vi "MLP_forwardpass_MLP2.vi"(11 "Array in":fxp<+/-,64,35>[](array[numeric])=[0.0, 0.0, 0.0, 0.0, 0.0, 0.0, 0.0, 0.0, 0.0, 0.0]) -> (3 "Numeric":fxp<+/-,32,16>)   [LabVIEW 2020]
uses:
  <vilib>/rvi/DataTransferAndStorage/Container/Common/niFpgaContainerExecOnDevCompGetState.vi
  <vilib>/rvi/Emulation/niFpgaEmulationIsFPGAContextNoSignature.vi
  <vilib>/rvi/DataTransferAndStorage/Container/Common/niFpgaContainerGetUniqueNameForEmu.vi
  <vilib>/rvi/Memory/Memory_Emulation/niFpgaMemoryEmulationCacheClearOnFirstRun.vi
  <vilib>/rvi/Memory/Memory_Emulation/nirvimemoryEmulationManagerCache_MakeExclusive.vi
  <vilib>/rvi/Memory/Memory_Emulation/niFpgaMemoryEmulationValidateCache.vi
  <vilib>/rvi/Memory/Memory_Emulation/nirvimemoryEmulationManagerCache_InsertValue.vi
  <vilib>/Utility/error.llb/Clear Errors.vi
  <vilib>/rvi/Memory/Memory_Emulation/nirvimemoryEmulationManagerCache_ReleaseExclusive.vi
  <vilib>/rvi/Memory/Memory_Emulation/nirvimemoryEmulationManagerCache_GetValue.vi
  <vilib>/rvi/Memory/Memory_Emulation/nirvimemoryEmulationManagerCache_SetValue.vi
  <vilib>/rvi/Emulation/niFpgaProcessEmulError.vi
  <vilib>/rvi/Emulation/niFpgaSctlEmulationGetInTimedLoop.vi
  <vilib>/rvi/errors/nirviReportUnexpectedCaseInternalError (U32).vi
  <vilib>/rvi/Emulation/niFpgaSctlEmulationResourceMgr.vi
  <vilib>/rvi/DataTransferAndStorage/Container/XNode/niFpgaContainer.xnode
  <vilib>/rvi/DataTransferAndStorage/Register/Emulation/niFpgaRegisterEmulationRefIn.vi
  <vilib>/rvi/Memory/Memory_Emulation/niFpgaMemoryEmulationRefIn.vi
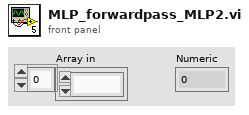
[diagram p1: front panel]
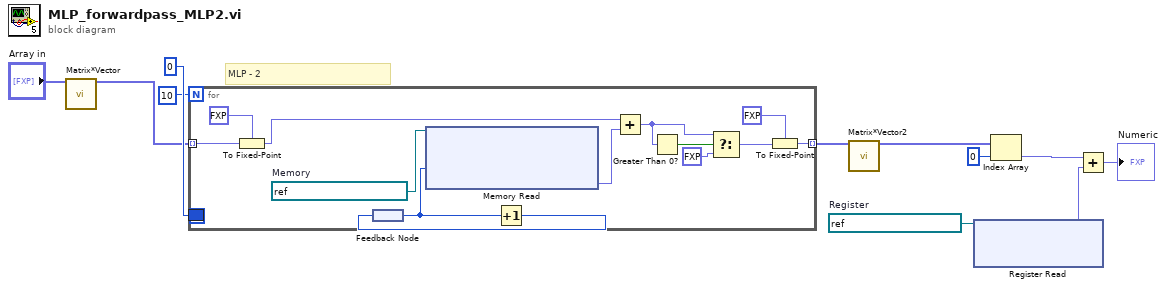
[diagram p0: block diagram]
diagram:
  w6 = refnum<k21> "Register-MLP_2_B_1"  # Register
  # "MLP - 2"
  n1 = call "Matrix*Vector"("Vector b"="Array in") -> ("Vector c"=w4:fxp<+/-,64,36>[])  [unwired: 10 in]
  n2 = for {
    N: 10 -> [_]
    tunnel: w4 -> [w15] mode=indexing
    tunnel: [w12] -> w3 mode=indexing
    border: u32 0 ("Timeout") -> [_]
    w19 = refnum<k21> "Memory-MLP_2_B_0"  # Memory
    n3 = To Fixed-Point(fixed-point type=fxp<+/-,32,16> 0.0 ("f"), number=w15) -> (fixed-point=w20:fxp<+/-,32,16>)
    n4 = feedback #1() -> (w18:u32)
    n5 = xnode ("Memory Read")("Address"=w18, "Memory In"=w19) -> ("Data"=w16:fxp<+/-,32,16>)  [unwired: 1 out]
    n6 = Increment(x=w18) -> (x+1=w17:u32)
    n7 = feedback-in #1(w17) -> ()
    n8 = Add(x=w20, y=w16) -> (x+y=w22:fxp<+/-,33,17>)
    n9 = Greater Than 0?(x=w22) -> (x > 0?=w24:bool)
    n10 = Select(t=w22, s=w24, f=fxp<+/-,33,17> 0.0) -> (s? t:f=w13:fxp<+/-,33,17>)
    n11 = To Fixed-Point(fixed-point type=fxp<+/-,32,16> 0.0 ("f"), number=w13) -> (fixed-point=w12:fxp<+/-,32,16>)
  }
  n12 = call "Matrix*Vector2"("Vector b"=w3) -> ("Vector c"=w5:fxp<+/-,64,36>[])  [unwired: 10 in]
  n13 = xnode ("Register Read")("Register In"=w6) -> ("Data"=w2:fxp<+/-,32,16>)  [unwired: 1 out]
  n14 = Index Array(array=w5, index=0) -> (element=w1:fxp<+/-,64,36>)
  n15 = Add(x=w1, y=w2) -> (x+y=→"Numeric":fxp<+/-,32,16>)
